vi "b2g1_sqlite_write_time.vi"(8 "error in (no error)":errorcluster, 9 "output cluster timestamp":timestamp, 10 "Database File":string, 11 "Output - Cluster b2g1":T1 {"TS-6 [°C]" format="%#.2g"; "TS-5 [°C]" format="%#.2g"; "pHS-1 [pH]" format="%.2g"; "TS-4 [°C]" format="%#.2g"; "FS-2 [l]" format="%.2g"; "FS-1 [l]" format="%.2g"; "DS-1 [bar]" format="%#.2g"; "DFS-1 [l/min]" format="%#.2g"; "FS-3 [l]" format="%.2g"; "DFS-1 [dl]" format="%.0g"}) -> (0 "error out":errorcluster)   [LabVIEW 2011]
uses:
  Output - Cluster b2g1.ctl
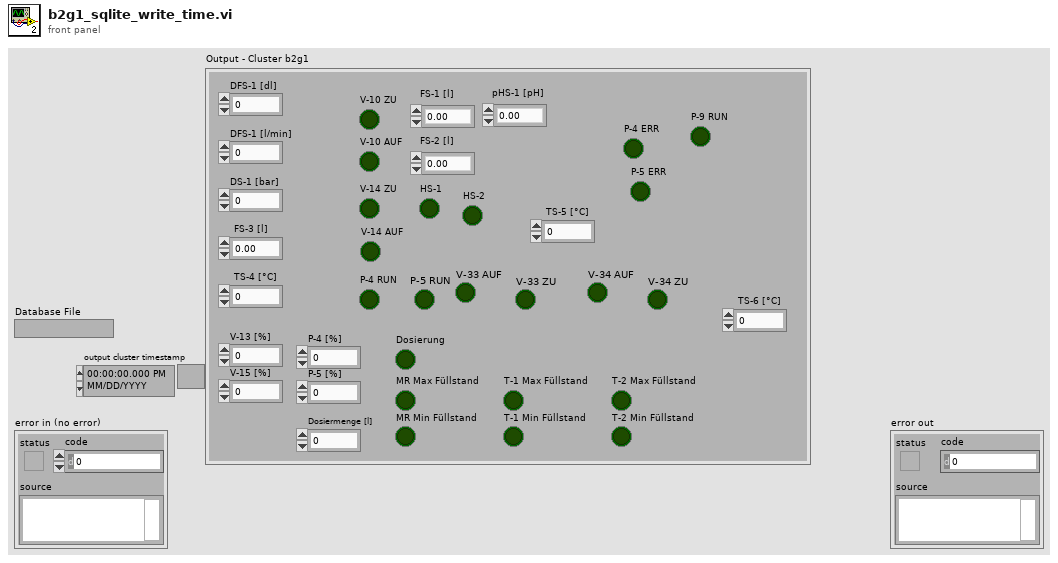
[diagram p1: front panel]
types:
  T1 = typedef "Output - Cluster b2g1.ctl" = cluster{"DFS-1 [dl]":u64, "FS-3 [l]":dbl, "DFS-1 [l/min]":dbl, "DS-1 [bar]":dbl, "V-10 ZU":bool, "V-14 ZU":bool, "FS-1 [l]":dbl, "FS-2 [l]":dbl, "TS-4 [°C]":dbl, "HS-1":bool, "V-13 [%]":u8, "V-15 [%]":u8, "P-4 [%]":u8, "P-5 [%]":u8, "Dosierung":bool, "MR Max Füllstand":bool, "MR Min Füllstand":bool, "Dosiermenge [l]":sgl, "V-14 AUF":bool, "V-10 AUF":bool, "T-1 Max Füllstand":bool, "T-1 Min Füllstand":bool, "T-2 Max Füllstand":bool, "T-2 Min Füllstand":bool, "pHS-1 [pH]":dbl, "P-4 RUN":bool, "P-5 RUN ":bool, "V-33 AUF":bool, "V-33 ZU":bool, "V-34 AUF":bool, "V-34 ZU":bool, "P-4 ERR":bool, "P-5 ERR":bool, "TS-5 [°C]":dbl, "TS-6 [°C]":dbl, "P-9 RUN":bool, "HS-2":bool}
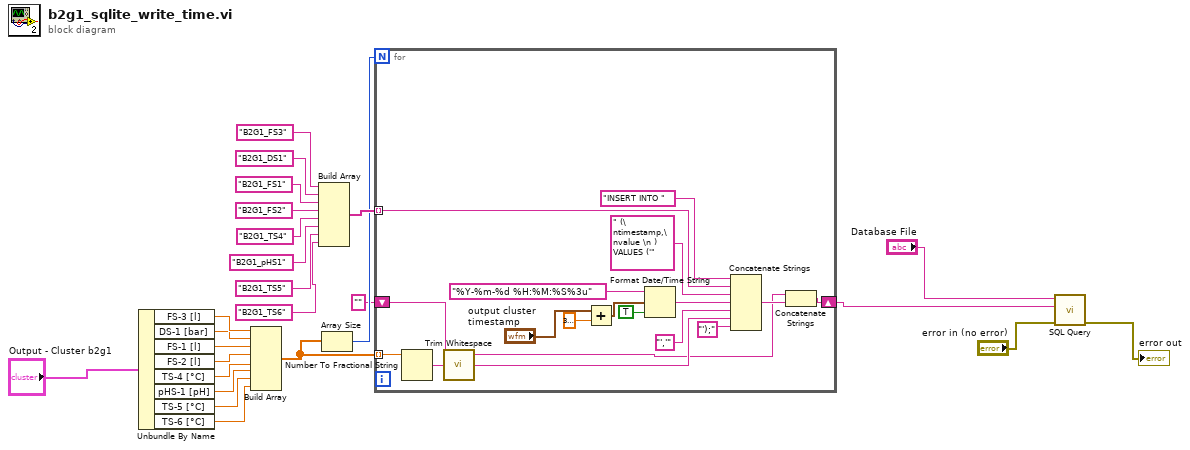
[diagram p0: block diagram]
diagram:
  n1 = Unbundle By Name("Output - Cluster b2g1") -> ("FS-3 [l]"=w25:dbl, "DS-1 [bar]"=w24:dbl, "FS-1 [l]"=w23:dbl, "FS-2 [l]"=w22:dbl, "TS-4 [°C]"=w21:dbl, "pHS-1 [pH]"=w20:dbl, "TS-5 [°C]"=w19:dbl, "TS-6 [°C]"=w2:dbl)
  n2 = Build Array(w25, w24, w23, w22, w21, w20, w19, w2) -> (w10:dbl[])
  n3 = Build Array("B2G1_FS3" ("SQL Query"), "B2G1_DS1" ("SQL Query"), "B2G1_FS1" ("SQL Query"), "B2G1_FS2" ("SQL Query"), "B2G1_TS4" ("SQL Query"), "B2G1_pHS1" ("SQL Query"), "B2G1_TS5" ("SQL Query"), "B2G1_TS6" ("SQL Query")) -> (w11:string[])
  n4 = Array Size(array=w10) -> (size(s)=w9:i32)
  n5 = for {
    N: w9 -> [_]
    tunnel: w10 -> [w33] mode=indexing
    tunnel: w11 -> [w32] mode=indexing
    shift-right: [w30] -> w6
    shift-left: "" -> [w29]
    n6 = Number To Fractional String(number=w33) -> (F-format string=w40:string)  [unwired: 3 in]
    n7 = call <vilib>:"Trim Whitespace.vi"("string"=w40) -> ("trimmed string"=w41:string)  [unwired: 1 in]
    n8 = Add(x="output cluster timestamp", y=dbl[unit] 3600.0) -> (x+y=w27:timestamp)
    n9 = Format Date/Time String(time format string (%c)="%Y-%m-%d %H:%M:%S%3u", seconds (now)=w27, UTC format=TRUE) -> (date/time string=w38:string)
    n10 = Concatenate Strings("INSERT INTO " ("SQL Query"), w32, " (\ntimestamp,\nvalue \n ) VALUES ('" ("SQL Query"), w38, "','" ("string"), w41, "');" ("string")) -> (w31:string)
    n11 = Concatenate Strings(w29, w31) -> (w30:string)
  }
  n12 = call "SQL Query.vi"("error in (no error)"="error in (no error)", "SQL Query"=w6, "Database File"="Database File") -> ("error out"=→"error out":errorcluster)  [unwired: 6 in, 2 out]
